vi "Test Client to Server.vi"(0 "Ports to Check":T4, 1 "Connection Established?":bool, 3 "error in (no error)":errorcluster) -> (7 "Results":T1, 8 "Test Finished?":bool, 10 "error out":errorcluster)   [LabVIEW 2019]
doc: "Tests ports in direction of cliend to server"
uses:
  controls/Ports to Check.ctl
  controls/Results.ctl
  controls/Log Data Cluster.ctl
  controls/Communication Types.ctl
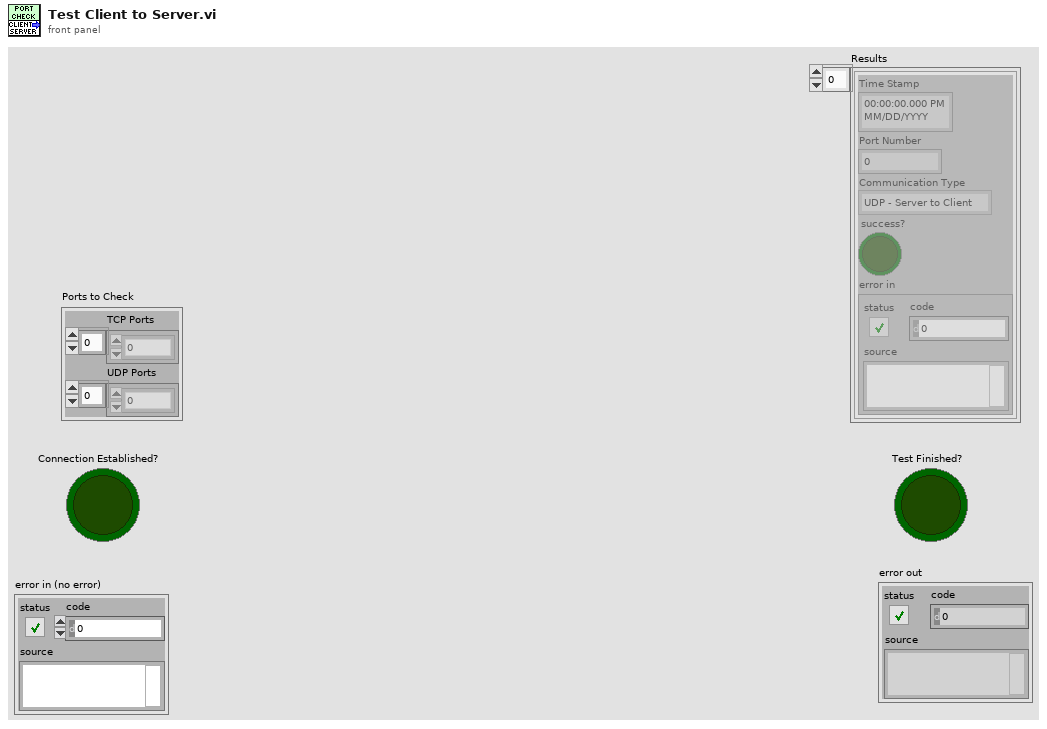
[diagram p1: front panel]
types:
  T1 = typedef "Results.ctl" = T2[]
  T2 = typedef "log data cluster.ctl" = cluster{"Time Stamp":timestamp, "Port Number":u16, "Communication Type":T3, "success?":bool, "error in":errorcluster}
  T3 = typedef "Communication Types.ctl" = enum16{"UDP - Server to Client", "UDP - Client to Server", "TCP - Server to Client", "TCP - Client to Server"}
  T4 = typedef "Ports to Check.ctl" = cluster{"TCP Ports":u16[], "UDP Ports":u16[]}
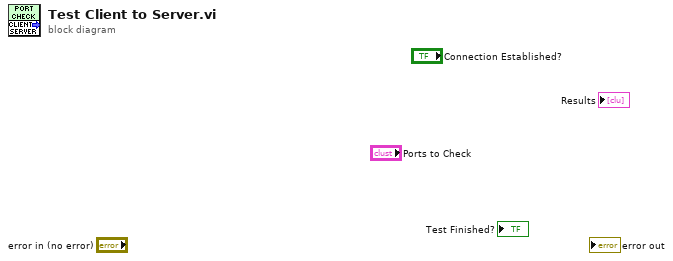
[diagram p0: block diagram]
diagram:
